vi "Send Log Data.vi"(8 "error in":errorcluster, 10 "Data":T2[](array[typedef]), 11 "Log Producer in":T1) -> (0 "error out":errorcluster, 3 "Log Producer out":T1)   [LabVIEW 2020, in "Frame Logging.lvlib"]
uses:
  Frame Logging.lvlib
  Shared/Frame.ctl
  Log_Producer.ctl
  Message_Request.ctl
  Message_Request_Action.ctl
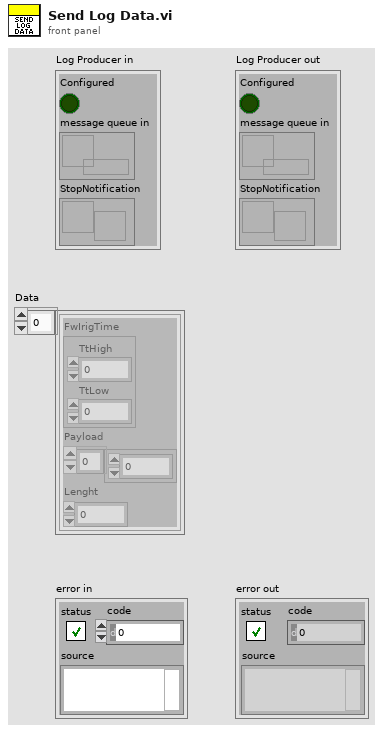
[diagram p1: front panel]
types:
  T1 = typedef "Frame Logging.lvlib/Log_Producer.ctl" = cluster{"Configured":bool, "message queue in":refnum<queue>, "StopNotification":refnum<notifier>}
  T2 = typedef "Frame.ctl" = cluster{"FwIrigTime":cluster{"TtHigh":u32, "TtLow":u32}, "Payload":u8[], "Lenght":u32}
  T3 = typedef "Frame Logging.lvlib/Message_Request_Action.ctl" = enum16{"Initialize", "Open File", "Log", "Manage Disk", "Stop", "Close File", "Update Configuration"}
  T4 = typedef "Frame Logging.lvlib/Message_Request.ctl" = cluster{"request":T3, "data":variant}
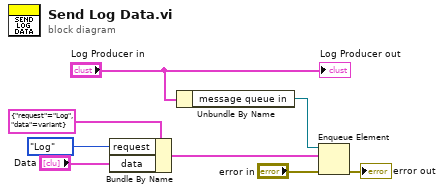
[diagram p0: block diagram]
diagram:
  n1 = Bundle By Name(cluster=T4 {"request"=enum."Log", "data"=variant} ("Message_type"), "request"=Message_Request_Action."Log", "data"="Data") -> (w6:T4)
  n2 = Unbundle By Name("Log Producer in") -> ("message queue in"=w7:refnum<queue>)
  n3 = Enqueue Element(queue=w7, element=w6, error in (no error)="error in") -> (error out=→"error out":errorcluster)  [unwired: 1 in, 2 out]
  "Log Producer out" <- "Log Producer in"
